vi "Multistaking.vi"() -> ()   [LabVIEW 2012]
doc: "M. Ferrari 18-5-1998 Multitasking function"
panel:
  in  "stop in":bool=TRUE
  in  "stop out":bool=TRUE
  in  "IN RATE (Hz)":dbl(knob)=1.0 scale=0.0..10.0 scale format="%.1f"
  in  "OUT RATE (Hz)":dbl(knob)=1.0 scale=0.0..10.0 scale format="%.1f"
  out "in waveform":dbl(graph)
  out "out waveform":dbl(graph)
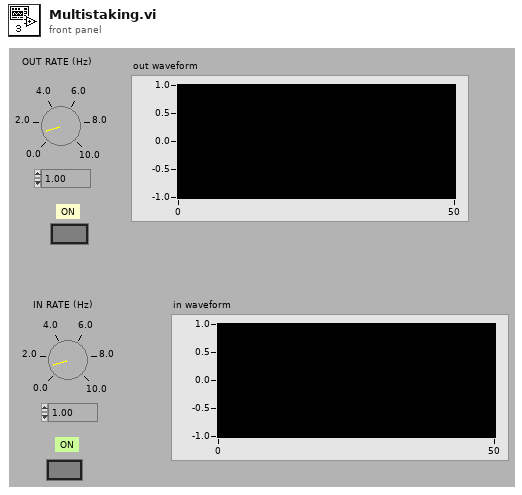
[diagram p1: front panel]
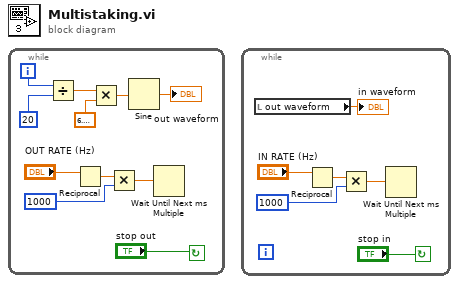
[diagram p0: block diagram]
diagram:
  n1 = while {
    i -> [w6]
    stop <- "stop out" continue-if-true
    n2 = Divide(x=w6, y=20) -> (x/y=w4:dbl)
    n3 = Reciprocal(x="OUT RATE (Hz)") -> (1/x=w9:dbl)
    n4 = Multiply(x=w4, y=6.283185307179586) -> (x*y=w2:dbl)
    n5 = Multiply(x=w9, y=1000) -> (x*y=w7:dbl)
    n6 = Sine(x=w2) -> (sin(x)=→"out waveform":dbl)
    n7 = Wait Until Next ms Multiple(millisecond multiple=w7) -> ()  [unwired: 1 out]
  }
  n8 = while {
    stop <- "stop in" continue-if-true
    n9 = local read "out waveform"() -> (→"in waveform":dbl)
    n10 = Reciprocal(x="IN RATE (Hz)") -> (1/x=w16:dbl)
    n11 = Multiply(x=w16, y=1000) -> (x*y=w14:dbl)
    n12 = Wait Until Next ms Multiple(millisecond multiple=w14) -> ()  [unwired: 1 out]
  }
